vi "簇的按名称捆绑与解绑.vi"() -> ()   [LabVIEW 2018]
panel:
  out "是否已经存在 2":bool
  out "位置 2":string
  out "名称 2":string
  out "编号 2":i32
  out "字符串":string="簇的捆绑与解除\n簇可以按名称捆绑或解除\n也可以不按名称捆绑或解除"
  in  "停止":bool
  out "输出簇":T1
  in  "是否已经存在":bool
  in  "位置":string
  in  "编号":i32
  in  "名称":string
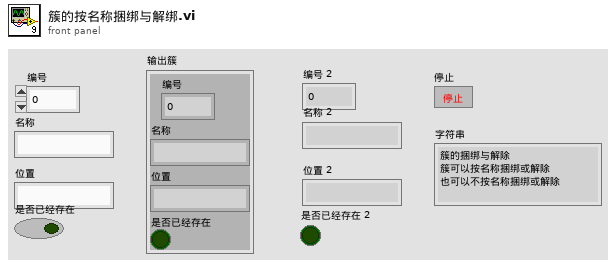
[diagram p1: front panel]
types:
  T1 = cluster{"编号":i32, "名称":string, "位置":string, "是否已经存在":bool}
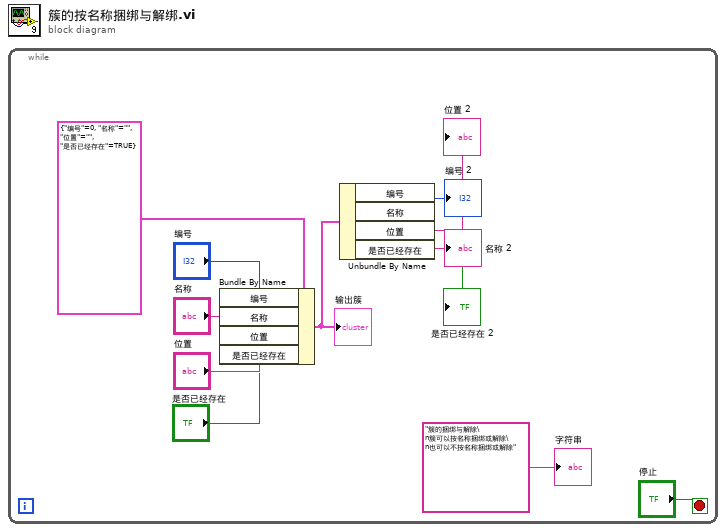
[diagram p0: block diagram]
diagram:
  n1 = while {
    stop <- "停止" stop-if-true
    n2 = Bundle By Name(cluster=T1 {"编号"=0, "名称"="", "位置"="", "是否已经存在"=TRUE} ("输入簇"), "编号"="编号", "名称"="名称", "位置"="位置", "是否已经存在"="是否已经存在") -> (w5:T1)
    "输出簇" <- w5
    n3 = Unbundle By Name(w5) -> ("编号"=→"编号 2":i32, "名称"=→"名称 2":string, "位置"=→"位置 2":string, "是否已经存在"=→"是否已经存在 2":bool)
    "字符串" <- "簇的捆绑与解除\n簇可以按名称捆绑或解除\n也可以不按名称捆绑或解除"
  }
